vi "Check For DBL Equality.vi"(3 "n2":dbl format="%0.17f", 4 "n1":dbl format="%0.17f") -> (1 "equal?":bool)   [LabVIEW 2015, in "Waveform Receive.lvclass"]
doc: "Check two floating point numbers for equality. Equality is defined as equal to 6 orders of magnitude. When comparing two numbers which are supposed to be zero, if one is zero, the other must be 1E-6 or less to get equality. If both are non-zero, they are compared as usual. This may cause errors for two numbers supposed to be zero, but with round-off error so they are not zero."
uses:
  Waveform Receive.lvclass
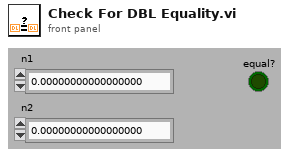
[diagram p1: front panel]
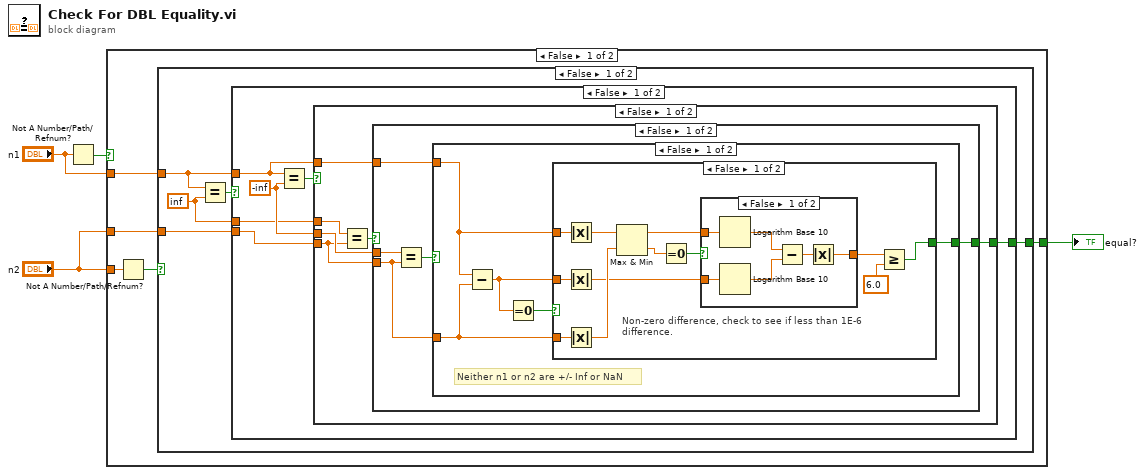
[diagram p0: block diagram]
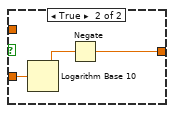
[diagram p2: hidden frame]
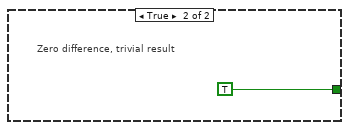
[diagram p3: hidden frame]
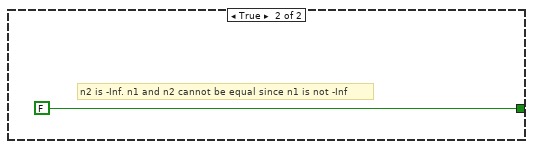
[diagram p4: hidden frame]
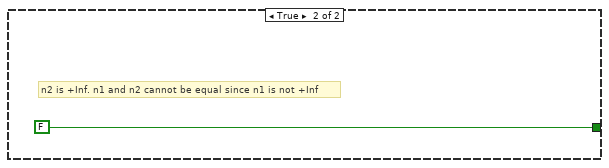
[diagram p5: hidden frame]
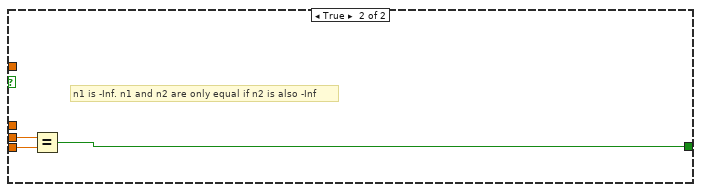
[diagram p6: hidden frame]
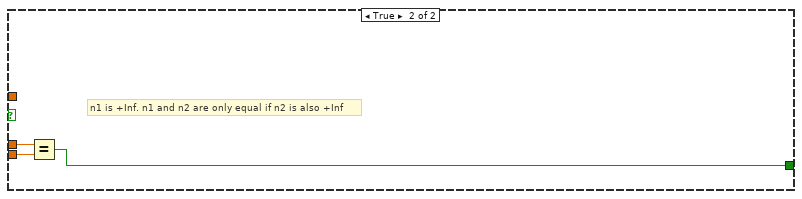
[diagram p7: hidden frame]
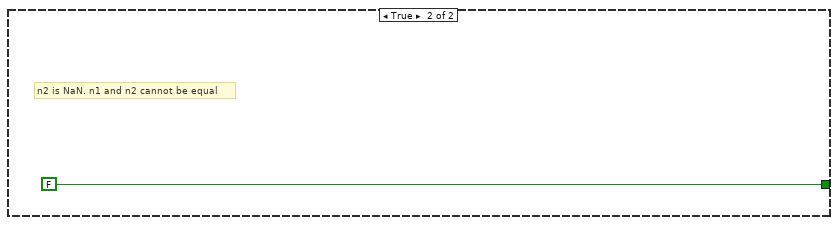
[diagram p8: hidden frame]
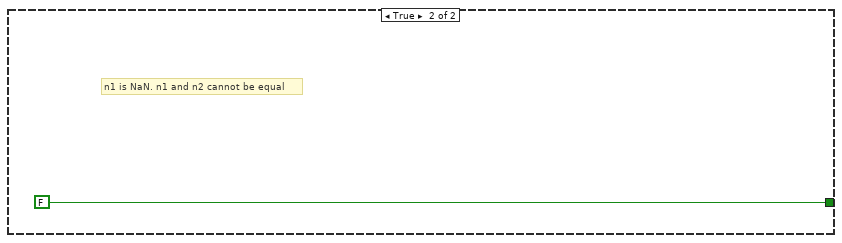
[diagram p9: hidden frame]
diagram:
  n1 = Not A Number/Path/Refnum?(number/path/refnum="n1") -> (NaN/Path/Refnum?=w4:bool)
  n2 = case shown="False" w4 {
    tunnel: [w7 FALSE] -> w3
    tunnel: "n2" -> [w9 _]
    tunnel: "n1" -> [w6 _]
    tunnel: "n2" -> [w5 _]
    frame False {
      n3 = Not A Number/Path/Refnum?(number/path/refnum=w9) -> (NaN/Path/Refnum?=w8:bool)
      n4 = case shown="False" w8 {
        tunnel: [w11 FALSE] -> w7
        tunnel: w6 -> [w10 _]
        tunnel: w5 -> [w13 _]
        frame False {
          w12 = inf
          n5 = Equal?(x=w10, y=w12) -> (x = y?=w14:bool)
          n6 = case shown="False" w14 {
            tunnel: w13 -> [w18 w66]
            tunnel: w12 -> [w16 w65]
            tunnel: [w17 w64] -> w11
            tunnel: w10 -> [w15 _]
            frame False {
              w19 = -inf
              n7 = Equal?(x=w15, y=w19) -> (x = y?=w20:bool)
              n8 = case shown="False" w20 {
                tunnel: w19 -> [w23 w63]
                tunnel: w18 -> [w22 w62]
                tunnel: [w24 w61] -> w17
                tunnel: w16 -> [w26 _]
                tunnel: w15 -> [w21 _]
                frame False {
                  n9 = Equal?(x=w26, y=w22) -> (x = y?=w25:bool)
                  n10 = case shown="False" w25 {
                    tunnel: [w29 FALSE] -> w24
                    tunnel: w23 -> [w31 _]
                    tunnel: w22 -> [w28 _]
                    tunnel: w21 -> [w27 _]
                    frame False {
                      n11 = Equal?(x=w31, y=w28) -> (x = y?=w30:bool)
                      n12 = case shown="False" w30 {
                        tunnel: [w32 FALSE] -> w29
                        tunnel: w28 -> [w34 _]
                        tunnel: w27 -> [w33 _]
                        frame False {
                          # "Neither n1 or n2 are +/- Inf or NaN"
                          n13 = Subtract(x=w33, y=w34) -> (x-y=w35:dbl)
                          n14 = Equal To 0?(x=w35) -> (x = 0?=w36:bool)
                          n15 = case shown="False" w36 {
                            tunnel: w35 -> [w48 _]
                            tunnel: w33 -> [w44 _]
                            tunnel: w34 -> [w43 _]
                            tunnel: [w45 TRUE] -> w32
                            frame False {
                              # "Non-zero difference, check to see if less than 1E-6 difference."
                              n16 = Absolute Value(x=w44) -> (abs(x)=w42:dbl)
                              n17 = Absolute Value(x=w48) -> (abs(x)=w39:dbl)
                              n18 = Absolute Value(x=w43) -> (abs(x)=w41:dbl)
                              n19 = Max & Min(x=w42, y=w41) -> (max(x,y)=w37:dbl, min(x,y)=w38:dbl)
                              n20 = Equal To 0?(x=w38) -> (x = 0?=w40:bool)
                              n21 = case shown="False" w40 {
                                tunnel: [w49 w55] -> w46
                                tunnel: w37 -> [w51 _]
                                tunnel: w39 -> [w50 w57]
                                frame False {
                                n22 = Logarithm Base 10(1:w51) -> (0:w54:dbl)
                                n23 = Logarithm Base 10(1:w50) -> (0:w53:dbl)
                                n24 = Subtract(x=w54, y=w53) -> (x-y=w52:dbl)
                                n25 = Absolute Value(x=w52) -> (abs(x)=w49:dbl)
                                }
                                frame True {
                                n26 = Logarithm Base 10(1:w57) -> (0:w56:dbl)
                                n27 = Negate(x=w56) -> (-x=w55:dbl)
                                }
                              }
                              n28 = Greater Or Equal?(x=w46, y=6.0) -> (x >= y?=w45:bool)
                            }
                            frame True {
                              # "Zero difference, trivial result"
                            }
                          }
                        }
                        frame True {
                          # "n2 is -Inf. n1 and n2 cannot be equal since n1 is not -Inf"
                        }
                      }
                    }
                    frame True {
                      # "n2 is +Inf. n1 and n2 cannot be equal since n1 is not +Inf"
                    }
                  }
                }
                frame True {
                  # "n1 is -Inf. n1 and n2 are only equal if n2 is also -Inf"
                  n29 = Equal?(x=w63, y=w62) -> (x = y?=w61:bool)
                }
              }
            }
            frame True {
              # "n1 is +Inf. n1 and n2 are only equal if n2 is also +Inf"
              n30 = Equal?(x=w65, y=w66) -> (x = y?=w64:bool)
            }
          }
        }
        frame True {
          # "n2 is NaN. n1 and n2 cannot be equal"
        }
      }
    }
    frame True {
      # "n1 is NaN. n1 and n2 cannot be equal"
    }
  }
  "equal?" <- w3
